vi "Calculate baseplate center.vi"() -> ()   [LabVIEW 2016]
panel:
  out "x-y 3":dbl
  out "theta 3":dbl
  out "x-y 2":dbl
  out "x-y":dbl
  out "theta 2":dbl
  out "r":dbl
  out "x/y 3":dbl[](array[numeric])
  out "x/y 2":dbl[](array[numeric])
  out "theta":dbl
  in  "array 2":dbl[][](array[numeric])
  out "x/y":dbl
  in  "array":dbl[][](array[numeric])
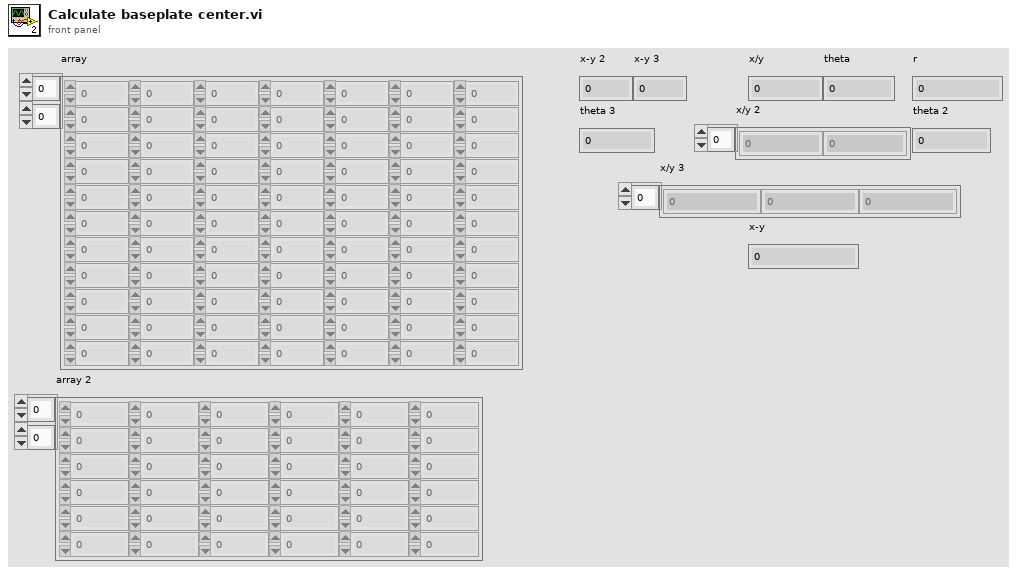
[diagram p1: front panel]
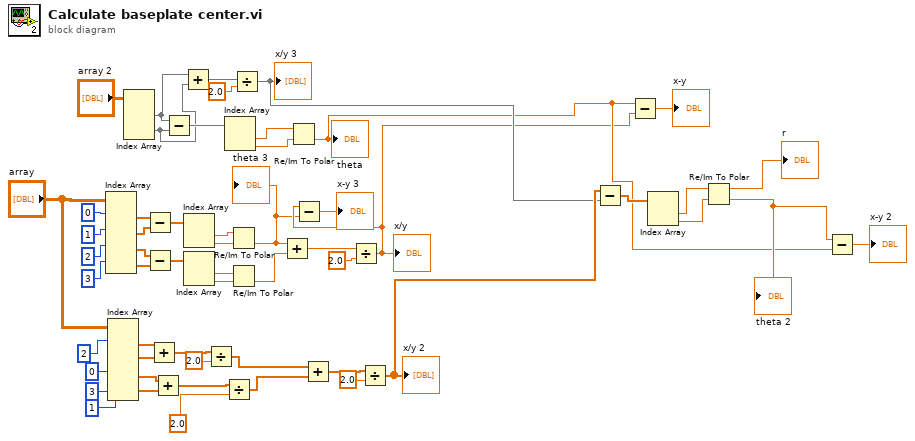
[diagram p0: block diagram]
diagram:
  n1 = Index Array(array="array", index (row) #1=0 ("index (row)"), index (row) #2=1 ("index (row)"), index (row) #3=2 ("index (row)"), index (row) #4=3 ("index (row)")) -> (element #1=w6:dbl[], element #2=w5:dbl[], element #3=w48:dbl[], element #4=w47:dbl[])  [unwired: 4 in]
  n2 = Index Array(array="array", index (row) #1=2 ("index (row)"), index (row) #2=0 ("index (row)"), index (row) #3=3 ("index (row)"), index (row) #4=1 ("index (row)")) -> (element #1=w35:dbl[], element #2=w34:dbl[], element #3=w33:dbl[], element #4=w32:dbl[])  [unwired: 4 in]
  n3 = Index Array(array="array 2") -> (element #1=w20:dbl[], element #2=w19:dbl[])  [unwired: 4 in]
  n4 = Subtract(x=w6, y=w5) -> (x-y=w46:dbl[])
  n5 = Subtract(x=w48, y=w47) -> (x-y=w45:dbl[])
  n6 = Add(x=w35, y=w34) -> (x+y=w31:dbl[])
  n7 = Add(x=w33, y=w32) -> (x+y=w28:dbl[])
  n8 = Subtract(x=w20, y=w19) -> (x-y=w40:dbl[])
  n9 = Add(x=w20, y=w19) -> (x+y=w18:dbl[])
  n10 = Index Array(array=w46) -> (element #1=w4:dbl, element #2=w44:dbl)  [unwired: 2 in]
  n11 = Index Array(array=w45) -> (element #1=w43:dbl, element #2=w42:dbl)  [unwired: 2 in]
  n12 = Divide(x=w31, y=2.0) -> (x/y=w25:dbl[])
  n13 = Divide(x=w28, y=2.0) -> (x/y=w24:dbl[])
  n14 = Index Array(array=w40) -> (element #1=w39:dbl, element #2=w38:dbl)  [unwired: 2 in]
  n15 = Re/Im To Polar(2:w44, 3:w4) -> (0:w2:dbl)  [unwired: 1 out]
  "theta 3" <- w2
  n16 = Re/Im To Polar(2:w42, 3:w43) -> (0:w55:dbl)  [unwired: 1 out]
  n17 = Divide(x=w18, y=2.0) -> (x/y=w14:dbl[])
  "x/y 3" <- w14
  n18 = Add(x=w2, y=w55) -> (x+y=w54:dbl)
  n19 = Re/Im To Polar(2:w38, 3:w39) -> (0:w8:dbl)  [unwired: 1 out]
  "theta" <- w8
  n20 = Add(x=w25, y=w24) -> (x+y=w27:dbl[])
  n21 = Divide(x=w54, y=2.0) -> (x/y=w3:dbl)
  "x/y" <- w3
  n22 = Subtract(x=w3, y=w2) -> (x-y=→"x-y 3":dbl)
  n23 = Divide(x=w27, y=2.0) -> (x/y=w15:dbl[])
  "x/y 2" <- w15
  n24 = Subtract(x=w15, y=w14) -> (x-y=w13:dbl[])
  n25 = Subtract(x=w8, y=w3) -> (x-y=→"x-y":dbl)
  n26 = Index Array(array=w13) -> (element #1=w12:dbl, element #2=w11:dbl)  [unwired: 2 in]
  n27 = Re/Im To Polar(2:w11, 3:w12) -> (0:w9:dbl, 1:→"r":dbl)
  "theta 2" <- w9
  n28 = Subtract(x=w9, y=w8) -> (x-y=→"x-y 2":dbl)
